vi "CCE RRMA P03 SubVI08.vi"(5 "Image 3":T1, 7 "NORMALIZACIÓN":bool, 8 "INVERTIDO?":bool, 9 "UMBRAL":u8(knob) scale=0.0..255.0, 10 "CAPA DE COLOR":T2(ring), 11 "Image":T1) -> (2 "MOMENTOS INVARIANTES DE HU":dbl[](array[numeric]), 3 "Image 2":T1)   [LabVIEW 2020]
doc: "Ceballos Conde Emanuel Rodríguez Ramírez Miguel Ángel 4MV6 Sistemas de visión artificial 2022/1\nEste vi permite obtener una imagen binarizada y LOS SIETE MOMENTOS INVARIANTES DE HU de una imagen, tomando como referencia una de las capas seleccionadas."
uses:
  <vilib>/vision/Image Controls.llb/IMAQ Image.ctl
panel:
  # "Ceballos Conde Emanuel\nRodríguez Ramírez Miguel Ángel\n4MV6\nSistemas de visión artificial\n2022/1"
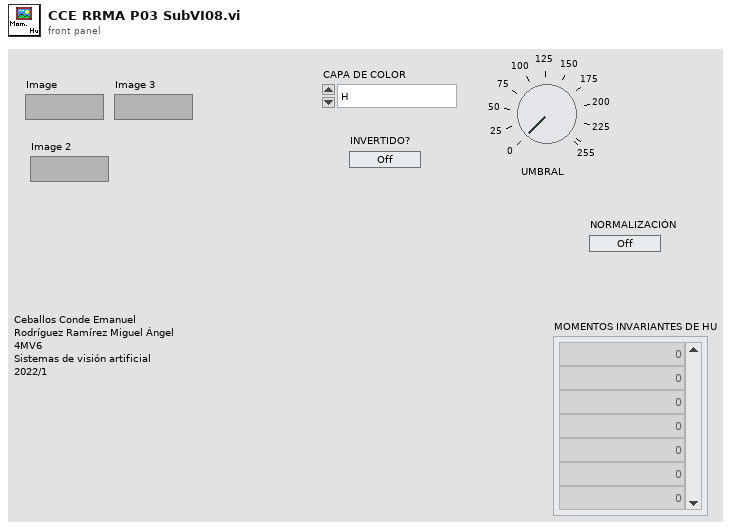
[diagram p1: front panel]
types:
  T1 = typedef "IMAQ Image.ctl" = refnum<image>
  T2 = enum16{"H", "S", "V", "C", "M", "Y", "R", "G", "B", "RGB2GRAY MATLAB"}
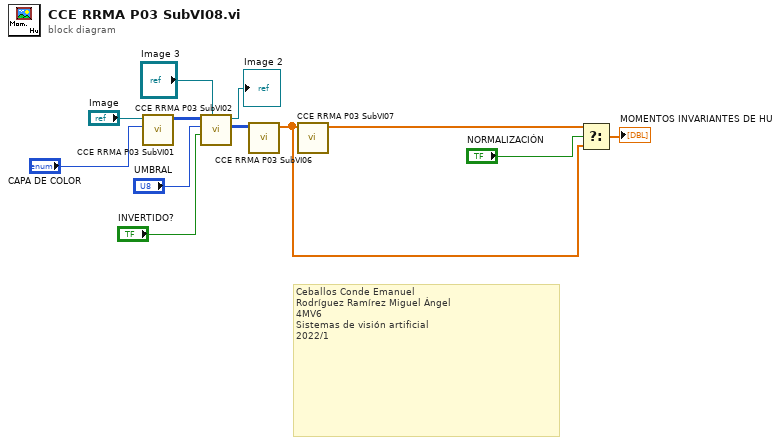
[diagram p0: block diagram]
diagram:
  # "Ceballos Conde Emanuel\nRodríguez Ramírez Miguel Ángel\n4MV6\nSistemas de visión artificial\n2022/1"
  n1 = call "CCE RRMA P03 SubVI01.vi"("CAPA DE COLOR"="CAPA DE COLOR", "Image"="Image") -> ("Array"=w4:u8[][])  [unwired: 9 in]
  n2 = call "CCE RRMA P03 SubVI02.vi"("Image"="Image 3", "INVERTIDO?"="INVERTIDO?", "UMBRAL"="UMBRAL", "Array"=w4) -> ("Array 2"=w5:u8[][], "Image Out"=→"Image 2":T1)  [unwired: 6 in]
  n3 = call "CCE RRMA P03 SubVI06.vi"("Image Data"=w5) -> ("HU"=w8:dbl[])  [unwired: 10 in]
  n4 = call "CCE RRMA P03 SubVI07.vi"("array"=w8) -> ("normalizado"=w9:dbl[])  [unwired: 10 in]
  n5 = Select(t=w9, s="NORMALIZACIÓN", f=w8) -> (s? t:f=→"MOMENTOS INVARIANTES DE HU":dbl[])
